vi "svx_Orbit Arrow.vi"(4 "shaft rotating direction":u16(ring) items=["CCW", "CW"], 6 "color":u32(colorbox)=10184, 9 "text max size":i16, 10 "Plot Area:Size":T1={"Width"=100, "Height"=100}, 11 "Picture in":picture) -> (2 "Plot Area:Size out":T1={"Width"=100, "Height"=100}, 3 "new picture":picture)   [LabVIEW 2017, in "SVX Orbit.xctl"]
uses:
  <vilib>/addons/_XControls/Orbit Plot/SVX Orbit.xctl
  <vilib>/Utility/miscctls.llb/LVBoundsTypeDef.ctl
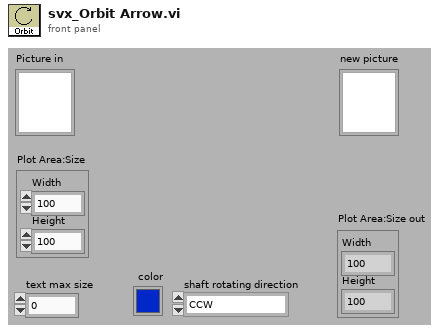
[diagram p1: front panel]
types:
  T1 = typedef "LVBoundsTypeDef.ctl" = cluster{"Width":u32, "Height":u32}
  T2 = cluster{"Width":u16, "Style":enum32{"Solid", "Dash", "Dot", "DashDot", "DashDotDot"}}
  T3 = cluster{"left":i16, "top":i16, "right":i16, "bottom":i16}
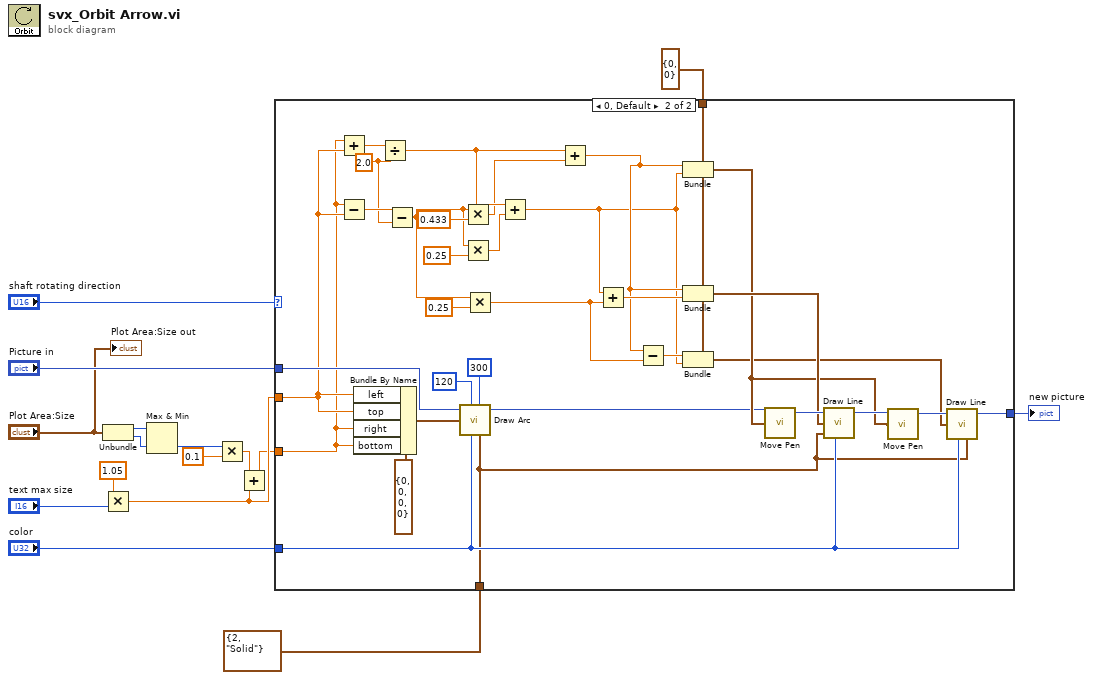
[diagram p0: block diagram]
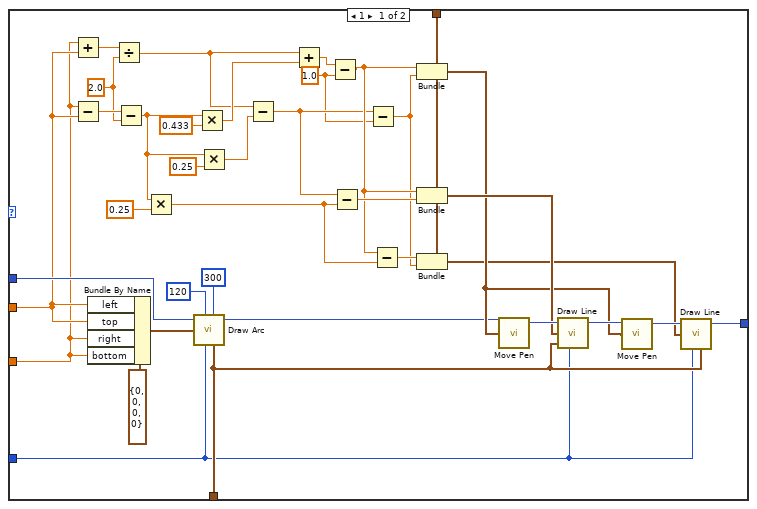
[diagram p2: hidden frame]
diagram:
  n1 = Unbundle("Plot Area:Size") -> ("Width"=w15:u32, "Height"=w14:u32)
  n2 = Multiply(x=1.05, y="text max size") -> (x*y=w4:dbl)
  n3 = Max & Min(x=w15, y=w14) -> (min(x,y)=w11:u32)  [unwired: 1 out]
  n4 = Multiply(x=w11, y=0.1) -> (x*y=w3:dbl)
  n5 = Add(x=w3, y=w4) -> (x+y=w2:dbl)
  n6 = case shown="0, Default" "shaft rotating direction" {
    tunnel: "Picture in" -> [w52 w85]
    tunnel: w2 -> [w34 w68]
    tunnel: w4 -> [w47 w80]
    tunnel: [w40 w73] -> w12
    tunnel: T2 {"Width"=2, "Style"=enum."Solid"} ("pen") -> [w38 w59]
    tunnel: "color" -> [w37 w71]
    tunnel: cluster{"x":i16, "y":i16} {"x"=0, "y"=0} ("cluster") -> [w17 w53]
    frame 1 {
      w21 = 1.0 ("y")
      w27 = 2.0 ("y")
      n7 = Add(x=w34, y=w47) -> (x+y=w36:dbl)
      n8 = Subtract(x=w34, y=w47) -> (x-y=w28:dbl)
      n9 = Bundle By Name(cluster=T3 {"left"=0, "top"=0, "right"=0, "bottom"=0} ("rect"), "left"=w47, "top"=w47, "right"=w34, "bottom"=w34) -> (w49:T3)
      n10 = Divide(x=w36, y=w27) -> (x/y=w26:dbl)
      n11 = Subtract(x=w28, y=w27) -> (x-y=w19:dbl)
      n12 = Multiply(x=w19, y=0.25) -> (x*y=w30:dbl)
      n13 = call <vilib>:"Draw Arc.vi"("picture"=w52, "start angle[degrees]"=i16 120, "rect"=w49, "color(black)"=w37, "arc size[degrees]"=i16 300, "pen"=w38) -> ("new picture"=w39:picture)  [unwired: 3 in]
      n14 = Multiply(x=w19, y=0.433) -> (x*y=w32:dbl)
      n15 = Multiply(x=w19, y=0.25) -> (x*y=w18:dbl)
      n16 = Subtract(x=w26, y=w18) -> (x-y=w23:dbl)
      n17 = Add(x=w26, y=w32) -> (x+y=w25:dbl)
      n18 = Subtract(x=w25, y=w21) -> (x-y=w24:dbl)
      n19 = Subtract(x=w23, y=w30) -> (x-y=w31:dbl)
      n20 = Subtract(x=w23, y=w21) -> (x-y=w22:dbl)
      n21 = Subtract(x=w24, y=w30) -> (x-y=w29:dbl)
      n22 = Bundle(cluster=w17, "x"=w24, "y"=w22) -> (w42:cluster{"x":i16, "y":i16})
      n23 = Bundle(cluster=w17, "x"=w24, "y"=w31) -> (w45:cluster{"x":i16, "y":i16})
      n24 = Bundle(cluster=w17, "x"=w29, "y"=w22) -> (w41:cluster{"x":i16, "y":i16})
      n25 = call <vilib>:"Move Pen.vi"("new position"=w42, "picture"=w39) -> ("new picture"=w46:picture)  [unwired: 3 in]
      n26 = call <vilib>:"Draw Line.vi"("picture"=w46, "end point"=w45, "color(black)"=w37, "pen"=w38) -> ("new picture"=w43:picture)  [unwired: 5 in]
      n27 = call <vilib>:"Move Pen.vi"("new position"=w42, "picture"=w43) -> ("new picture"=w44:picture)  [unwired: 3 in]
      n28 = call <vilib>:"Draw Line.vi"("picture"=w44, "end point"=w41, "color(black)"=w37, "pen"=w38) -> ("new picture"=w40:picture)  [unwired: 5 in]
    }
    frame 0, Default {
      w61 = 2.0 ("y")
      n29 = Add(x=w68, y=w80) -> (x+y=w70:dbl)
      n30 = Subtract(x=w68, y=w80) -> (x-y=w62:dbl)
      n31 = Bundle By Name(cluster=T3 {"left"=0, "top"=0, "right"=0, "bottom"=0} ("rect"), "left"=w80, "top"=w80, "right"=w68, "bottom"=w68) -> (w82:T3)
      n32 = Divide(x=w70, y=w61) -> (x/y=w67:dbl)
      n33 = Subtract(x=w62, y=w61) -> (x-y=w56:dbl)
      n34 = call <vilib>:"Draw Arc.vi"("picture"=w85, "start angle[degrees]"=i16 120, "rect"=w82, "color(black)"=w71, "arc size[degrees]"=i16 300, "pen"=w59) -> ("new picture"=w72:picture)  [unwired: 3 in]
      n35 = Multiply(x=w56, y=0.433) -> (x*y=w60:dbl)
      n36 = Multiply(x=w56, y=0.25) -> (x*y=w54:dbl)
      n37 = Multiply(x=w56, y=0.25) -> (x*y=w65:dbl)
      n38 = Add(x=w67, y=w54) -> (x+y=w57:dbl)
      n39 = Add(x=w67, y=w60) -> (x+y=w58:dbl)
      n40 = Add(x=w57, y=w65) -> (x+y=w66:dbl)
      n41 = Subtract(x=w58, y=w65) -> (x-y=w64:dbl)
      n42 = Bundle(cluster=w53, "x"=w58, "y"=w57) -> (w75:cluster{"x":i16, "y":i16})
      n43 = Bundle(cluster=w53, "x"=w58, "y"=w66) -> (w78:cluster{"x":i16, "y":i16})
      n44 = Bundle(cluster=w53, "x"=w64, "y"=w57) -> (w74:cluster{"x":i16, "y":i16})
      n45 = call <vilib>:"Move Pen.vi"("new position"=w75, "picture"=w72) -> ("new picture"=w79:picture)  [unwired: 3 in]
      n46 = call <vilib>:"Draw Line.vi"("picture"=w79, "end point"=w78, "color(black)"=w71, "pen"=w59) -> ("new picture"=w76:picture)  [unwired: 5 in]
      n47 = call <vilib>:"Move Pen.vi"("new position"=w75, "picture"=w76) -> ("new picture"=w77:picture)  [unwired: 3 in]
      n48 = call <vilib>:"Draw Line.vi"("picture"=w77, "end point"=w74, "color(black)"=w71, "pen"=w59) -> ("new picture"=w73:picture)  [unwired: 5 in]
    }
  }
  "new picture" <- w12
  "Plot Area:Size out" <- "Plot Area:Size"
